vi "Bridge Close.vi"(8 "error in":errorcluster, 11 "bridge in":T1={"type"=enum."TWM client", "TWM"={"pipe name"="", "parameters"=[], "handle"=0, "fixed aper [s]"=0.0, "f-list [Hz]"=[], "discrete f-list"=FALSE, "unc mode"=enum."None", "unc mcc"=0, "unc first"=FALSE}, "last f"=0.0, "bias comp"={"bias type"=enum."dummy", "VISA"="", "Enable"=FALSE, "channel qu"=[], "channel Uinit"=[]}, "sim mode"=enum."Generic RLC network", "channel idns"=[], "sim phases"=1} {"TWM"."f-list [Hz]" format="%#_6p"}) -> (0 "error out":errorcluster, 3 "bridge out":T1={"type"=enum."TWM client", "TWM"={"pipe name"="", "parameters"=[], "handle"=0, "fixed aper [s]"=0.0, "f-list [Hz]"=[], "discrete f-list"=FALSE, "unc mode"=enum."None", "unc mcc"=0, "unc first"=FALSE}, "last f"=0.0, "bias comp"={"bias type"=enum."dummy", "VISA"="", "Enable"=FALSE, "channel qu"=[], "channel Uinit"=[]}, "sim mode"=enum."Generic RLC network", "channel idns"=[], "sim phases"=1} {"TWM"."f-list [Hz]" format="%#_6p"})   [LabVIEW 2020]
doc: "Close bridge."
uses:
  Bridge Session.ctl
  Bridge Type.ctl
  drivers/TWM client/TWM Session.ctl
  drivers/TWM client/TWM parameters.ctl
  drivers/TWM client/Meas Proc QWTB Uncertainty Mode.ctl
  Bridge Bias Session.ctl
  Bridge Bias Type.ctl
  Bridge Sim Mode.ctl
  drivers/TWM client.lvlibp
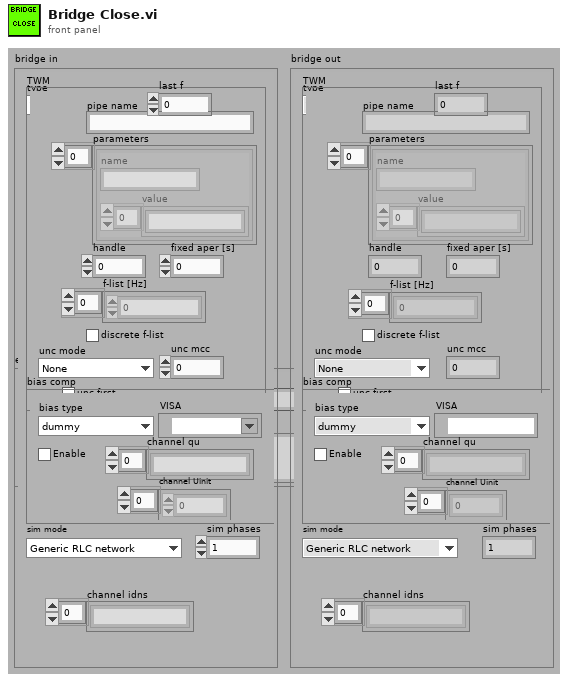
[diagram p1: front panel]
types:
  T1 = typedef "Bridge Session.ctl" = cluster{"type":T2, "TWM":T3, "last f":dbl, "bias comp":T6, "sim mode":T8, "channel idns":string[], "sim phases":i32}
  T2 = typedef "Bridge Type.ctl" = enum16{"TWM client", "dummy"}
  T3 = typedef "TWM Session.ctl" = cluster{"pipe name":string, "parameters":T4[], "handle":i32, "fixed aper [s]":dbl, "f-list [Hz]":dbl[], "discrete f-list":bool, "unc mode":T5, "unc mcc":i32, "unc first":bool}
  T4 = typedef "TWM parameters.ctl" = cluster{"name":string, "value":string[]}
  T5 = typedef "Meas Proc QWTB Uncertainty Mode.ctl" = enum16{"None", "GUF", "Monte Carlo"}
  T6 = typedef "Bridge Bias Session.ctl" = cluster{"bias type":T7, "VISA":refnum<visa-resource-name>, "Enable":bool, "channel qu":string[], "channel Uinit":dbl[]}
  T7 = typedef "Bridge Bias Type.ctl" = enum16{"dummy", "CMI LiBbias V1.0"}
  T8 = typedef "Bridge Sim Mode.ctl" = enum16{"Generic RLC network", "Interchannel transfer"}
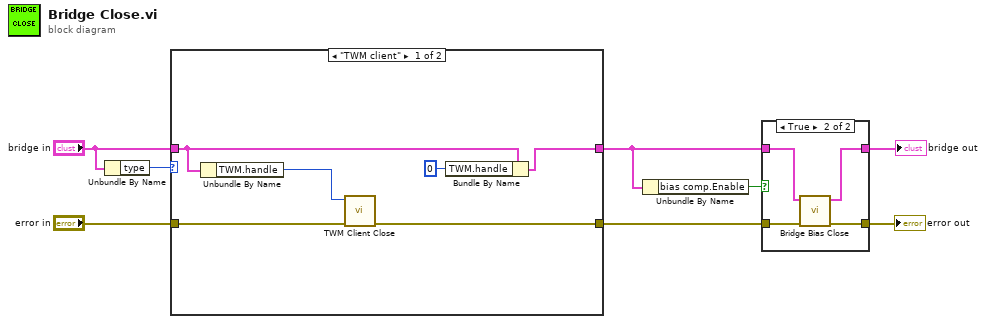
[diagram p0: block diagram]
diagram:
  n1 = Unbundle By Name("bridge in") -> ("type"=w8:T2)
  n2 = case shown="\"TWM client\"" w8 {
    tunnel: "error in" -> [w12 w16]
    tunnel: [w11 w16] -> w4
    tunnel: "bridge in" -> [w14 w15]
    tunnel: [w13 w15] -> w3
    frame "TWM client" {
      n3 = Unbundle By Name(w14) -> ("TWM.handle"=w10:i32)
      n4 = call "TWM Client Close.vi"("error in"=w12, "handle in"=w10) -> ("error out"=w11:errorcluster)  [unwired: 9 in]
      n5 = Bundle By Name(cluster=w14, "TWM.handle"=0) -> (w13:T1)
    }
    frame "dummy", Default {
    }
  }
  n6 = Unbundle By Name(w3) -> ("bias comp.Enable"=w5:bool)
  n7 = case shown="True" w5 {
    tunnel: w4 -> [w17 w22]
    tunnel: [w17 w21] -> w1
    tunnel: w3 -> [w18 w20]
    tunnel: [w18 w19] -> w2
    frame False {
    }
    frame True {
      n8 = call "Bridge Bias Close.vi"("error in"=w22, "bridge in"=w20) -> ("error out"=w21:errorcluster, "bridge out"=w19:T1)  [unwired: 8 in]
    }
  }
  "error out" <- w1
  "bridge out" <- w2
